vi "KE622x -- Set Display Params.vi"(0 "Resource In":refnum<visa-resource-name>, 1 "Check For SCPI Errors? (T)":bool=TRUE, 7 "Display Params":T1={"Display\nEnabled?"=TRUE, "Custom Top\nLine Text?"=FALSE, "Top Line Text (20 chars max)"="", "Custom Bottom\nLine Text?"=FALSE, "Bottom Line Text (32 chars max)"=""}, 11 "error in (no error)":errorcluster) -> (4 "Resource Out (dupl)":refnum<visa-resource-name>, 15 "error out":errorcluster)   [LabVIEW 2019, in "Keithley 622x.lvlib"]
doc: "Sets parameters for the KE622x front panel display."
uses:
  Keithley 622x.lvlib
  Typedefs/KE622x -- Display Params.ctl
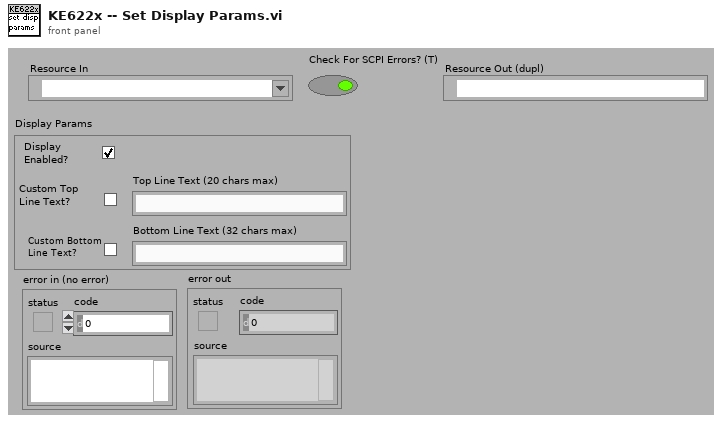
[diagram p1: front panel]
types:
  T1 = typedef "Keithley 622x.lvlib/KE622x -- Display Params.ctl" = cluster{"Display\nEnabled?":bool, "Custom Top\nLine Text?":bool, "Top Line Text (20 chars max)":string, "Custom Bottom\nLine Text?":bool, "Bottom Line Text (32 chars max)":string}
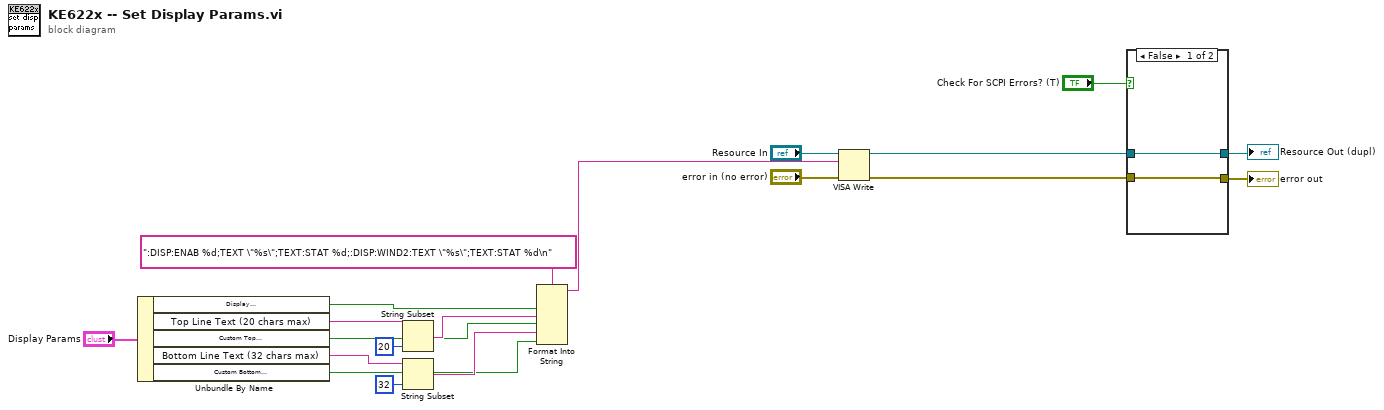
[diagram p0: block diagram]
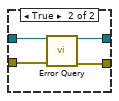
[diagram p2: hidden frame]
diagram:
  n1 = Unbundle By Name("Display Params") -> ("Display\nEnabled?"=w8:bool, "Top Line Text (20 chars max)"=w7:string, "Custom Top\nLine Text?"=w4:bool, "Bottom Line Text (32 chars max)"=w3:string, "Custom Bottom\nLine Text?"=w1:bool)
  n2 = String Subset(string=w7, length (rest)=20 ("length (rest)")) -> (substring=w5:string)  [unwired: 1 in]
  n3 = String Subset(string=w3, length (rest)=32 ("length (rest)")) -> (substring=w2:string)  [unwired: 1 in]
  n4 = Format Into String(format string=":DISP:ENAB %d;TEXT \"%s\";TEXT:STAT %d;:DISP:WIND2:TEXT \"%s\";TEXT:STAT %d\n", w8, w5, w4, w2, w1) -> (resulting string=w6:string)  [unwired: 2 in, 1 out]
  n5 = VISA Write(VISA resource name="Resource In", write buffer=w6, error in (no error)="error in (no error)") -> (VISA resource name out=w16:refnum<visa-resource-name>, error out=w15:errorcluster)  [unwired: 1 out]
  n6 = case shown="False" "Check For SCPI Errors? (T)" {
    tunnel: w16 -> [w21 w25]
    tunnel: w15 -> [w20 w24]
    tunnel: [w20 w23] -> w13
    tunnel: [w21 w22] -> w14
    frame False {
    }
    frame True {
      n7 = call "Error Query.vi"("VISA Resource In"=w25, "error in (no error)"=w24) -> ("VISA Resource Out (dupl)"=w22:refnum<visa-resource-name>, "error out"=w23:errorcluster)  [unwired: 10 in, 2 out]
    }
  }
  "Resource Out (dupl)" <- w14
  "error out" <- w13
